vi "AssertSubpanelExecState_Tests.vi"(11 "error in":errorcluster) -> (15 "error out":errorcluster)   [LabVIEW 2016, in "DronaTest.lvlib"]
uses:
  DronaTest.lvlib
  APIs/Stimulus/ControlValue/ValueSignalByPathString.vi
  APIs/Assert/AssertSubpanel/AssertSubpanelVIExecIdle.vi
  APIs/Stimulus/ControlValue/ValueSignalLatchBooleanString.vi
  APIs/Assert/AssertSubpanel/AssertSubpanelVIExecRunning.vi
  <vilib>/addons/_JKI Toolkits/Caraya/classes/Test/Test.lvclass
  Drona.lvlib
  APIs/Stimulus/ControlValue/ControlValue.lvlib
  <vilib>/addons/_JKI Toolkits/Caraya/classes/Assert/Assert.lvclass
  APIs/Assert/AssertSubpanel/AssertSubpanel.lvlib
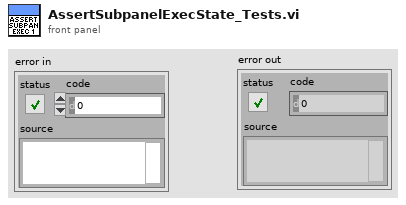
[diagram p1: front panel]
types:
  T1 = enum32{"Bad", "Idle", "Run top level", "Running"}
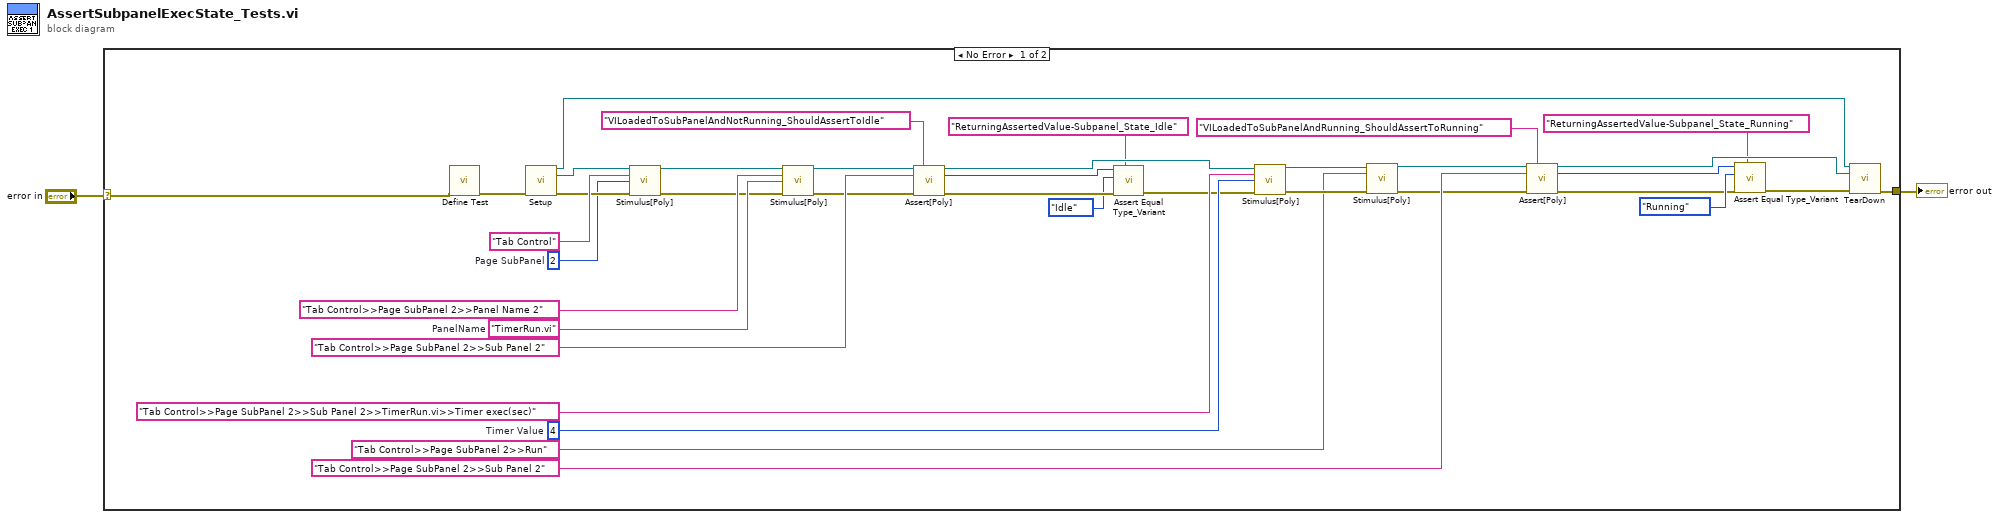
[diagram p0: block diagram]
diagram:
  n1 = case shown="No Error" "error in" {
    selector: "error in" -> [w38 w40]
    tunnel: [w21 w40] -> w1
    frame No Error {
      w28 = 4  # Timer Value
      w18 = 2  # Page SubPanel
      w34 = "TimerRun.vi"  # PanelName
      n2 = call <vilib>:"Define Test.vi"("error in (no error)"=w38) -> ("error out"=w32:errorcluster)  [unwired: 9 in, 1 out]
      n3 = call "Setup.vi"("error in (no error)"=w32) -> ("Application Ref"=w19:refnum<vi>, "VI out"=w20:refnum<vi>, "error out"=w22:errorcluster)  [unwired: 12 in]
      n4 = call-poly "Stimulus[Poly].vi"("VI Reference In"=w20, "Control Path"="Tab Control", "Value (Signaling)"=w18, "error in"=w22) -> ("VI Reference Out"=w33:refnum<vi>, "error out"=w30:errorcluster)  [unwired: 10 in]
      n5 = call-poly "Stimulus[Poly].vi"("VI Reference In"=w33, "Control Path"="Tab Control>>Page SubPanel 2>>Panel Name 2", "Value (Signaling)"=w34, "error in"=w30) -> ("VI Reference Out"=w17:refnum<vi>, "error out"=w16:errorcluster)  [unwired: 10 in]
      n6 = call-poly "Assert[Poly].vi"("VI Reference In"=w17, "Test Label"="VILoadedToSubPanelAndNotRunning_ShouldAssertToIdle" ("Label"), "Control Path"="Tab Control>>Page SubPanel 2>>Sub Panel 2", "Error In"=w16) -> ("VI Reference Out"=w15:refnum<vi>, "Asserted Value"=w10:T1, "Error Out"=w12:errorcluster)  [unwired: 9 in]
      n7 = call <vilib>:"Assert Equal Type_Variant.vi"("Label"="ReturningAssertedValue-Subpanel_State_Idle", "error in (no error)"=w12, "Y"=T1."Idle" ("Asserted Value"), "X"=w10) -> ("error out"=w11:errorcluster)  [unwired: 6 in, 1 out]
      n8 = call-poly "Stimulus[Poly].vi"("VI Reference In"=w15, "Control Path"="Tab Control>>Page SubPanel 2>>Sub Panel 2>>TimerRun.vi>>Timer exec(sec)", "Value (Signaling)"=w28, "error in"=w11) -> ("VI Reference Out"=w27:refnum<vi>, "error out"=w26:errorcluster)  [unwired: 10 in]
      n9 = call-poly "Stimulus[Poly].vi"("VI Reference In"=w27, "Control Path"="Tab Control>>Page SubPanel 2>>Run", "error in"=w26) -> ("VI Reference Out"=w24:refnum<vi>, "error out"=w23:errorcluster)  [unwired: 11 in]
      n10 = call-poly "Assert[Poly].vi"("VI Reference In"=w24, "Test Label"="VILoadedToSubPanelAndRunning_ShouldAssertToRunning" ("Label"), "Control Path"="Tab Control>>Page SubPanel 2>>Sub Panel 2", "Error In"=w23) -> ("VI Reference Out"=w13:refnum<vi>, "Asserted Value"=w3:T1, "Error Out"=w6:errorcluster)  [unwired: 9 in]
      n11 = call <vilib>:"Assert Equal Type_Variant.vi"("Label"="ReturningAssertedValue-Subpanel_State_Running", "error in (no error)"=w6, "Y"=T1."Running" ("Asserted Value"), "X"=w3) -> ("error out"=w5:errorcluster)  [unwired: 6 in, 1 out]
      n12 = call "TearDown.vi"("Application Ref"=w19, "VI in"=w13, "error in (no error)"=w5) -> ("error out"=w21:errorcluster)  [unwired: 12 in]
    }
    frame Error {
    }
  }
  "error out" <- w1
